vi "SECoP-addPropertyInteger.vi"(8 "error in (no error)":errorcluster, 9 "property value":i64, 10 "property name":string, 11 "DLL path (in)":T1) -> (0 "error out":errorcluster, 3 "DLL path (out)":T1)   [LabVIEW 2023, in "SECoP.lvlib"]
doc: "Call <b>\"SECoP-addPropertyInteger.vi\"</b> to append a SECoP integer property to the last SEC node, module, command or parameter. This is a convenience function like \"SECoP-addProperty.vi\" with an integer.\n\n<b>DLL path</b> input and output of cluster from \"SECoP-Initialize.vi\"\n<b>property name</b> name of property\n<b>property value</b> value of the property"
uses:
  SECoP.lvlib
  SECoP-libraries.ctl
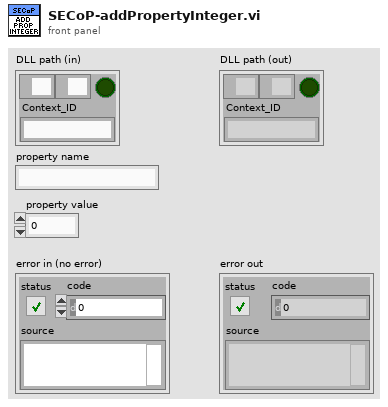
[diagram p1: front panel]
types:
  T1 = typedef "SECoP.lvlib/SECoP-libraries.ctl" = cluster{"serverDLL":path, "variantDLL":path, "cleanup_mode":bool, "Context_ID":string}
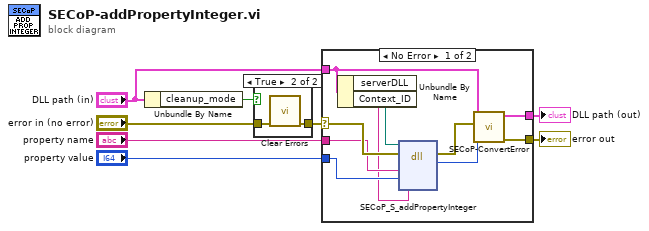
[diagram p0: block diagram]
diagram:
  n1 = Unbundle By Name("DLL path (in)") -> ("cleanup_mode"=w5:bool)
  n2 = case shown="True" w5 {
    tunnel: "error in (no error)" -> [w9 w11]
    tunnel: [w9 w10] -> w3
    frame False {
    }
    frame True {
      n3 = call <vilib>:"Clear Errors.vi"("error in (no error)"=w11) -> ("error out"=w10:errorcluster)  [unwired: 5 in, 1 out]
    }
  }
  n4 = case shown="No Error" w3 {
    selector: w3 -> [w18 w22]
    tunnel: "DLL path (in)" -> [w14 w23]
    tunnel: [w20 w23] -> w8
    tunnel: [w21 w22] -> w7
    tunnel: "property name" -> [w17 _]
    tunnel: "property value" -> [w16 _]
    frame No Error {
      n5 = Unbundle By Name(w14) -> ("serverDLL"=w13:path, "Context_ID"=w12:string)
      n6 = dll-call lib="Z:/Praktische Aufgaben/SECoP-LabVIEW2015/32bit/SECoP32.dll" fn="SECoP_S_addPropertyInteger"(path in=w13, error in=w18, "Name"=w17, "Value"=w16, "szContextID"=w12) -> (error out=w19:errorcluster, "return type"=w15:i32)  [unwired: 4 in, 1 out]
      n7 = call "SECoP-ConvertError.vi"("return code"=w15, "error in (no error)"=w19, "DLL path (in)"=w14) -> ("error out"=w21:errorcluster, "DLL path (out)"=w20:T1)  [unwired: 7 in]
    }
    frame Error {
    }
  }
  "DLL path (out)" <- w8
  "error out" <- w7
